vi "getSelectionValues.vi"(8 "error in (no error)":errorcluster, 11 "IProperty in":refnum<class "IProperty.lvclass">) -> (0 "error out":errorcluster, 2 "Selection Values out":refnum<class "IBaseObject.lvclass">, 3 "IProperty out":refnum<class "IProperty.lvclass">, 4 "Null?":bool)   [LabVIEW 2022 SP3, in "openDAQ.lvlib" / "IBaseObject.lvlib" / "IProperty.lvlib" / "IProperty.lvclass"]
uses:
  <instrlib>/openDAQ/Public/Classes/IProperty/IProperty.lvclass
  C:/Program Files (x86)/National Instruments/LabVIEW 2022/instr.lib/openDAQ/Public/Classes/IBaseObject/IBaseObject.lvclass
  <instrlib>/openDAQ/Public/Classes/IBaseObject/IBaseObject.lvclass
  <instrlib>/openDAQ/Public/Classes/IBaseObject/IBaseObject.lvclass/IBaseObject.ctl
  <instrlib>/openDAQ/Public/Classes/IBaseObject/Accessor/Read reference.vi
  <instrlib>/openDAQ/Public/Classes/IBaseObject/Accessor/Write reference.vi
  <instrlib>/openDAQ/Public/Classes/IProperty/IProperty.lvclass/IProperty.ctl
  <instrlib>/openDAQ/Binaries/Windows/x86/copendaq32.dll
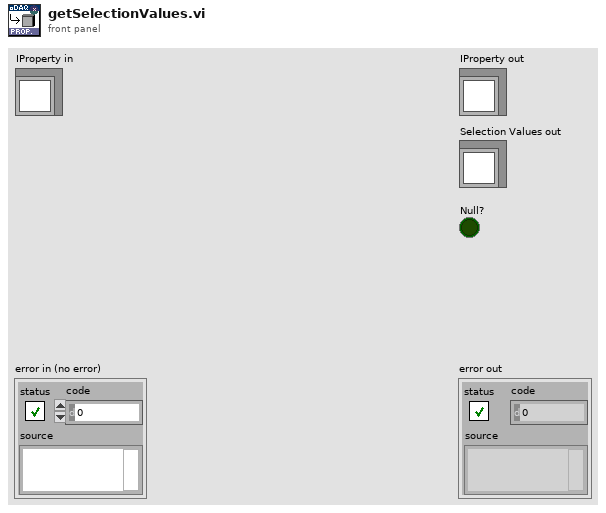
[diagram p1: front panel]
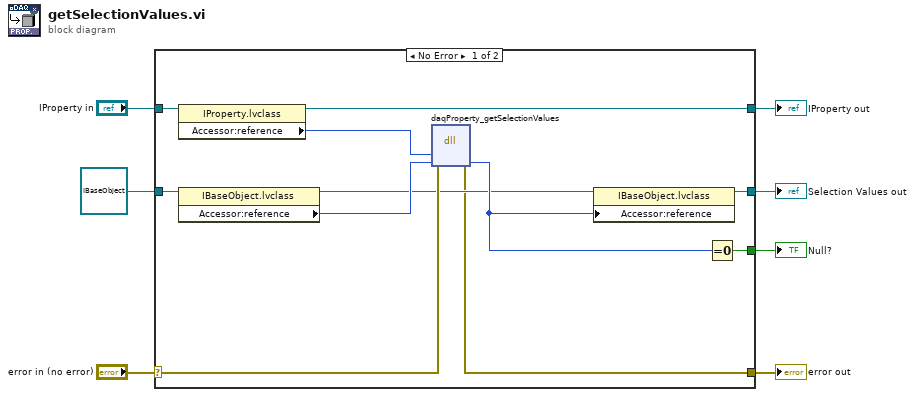
[diagram p0: block diagram]
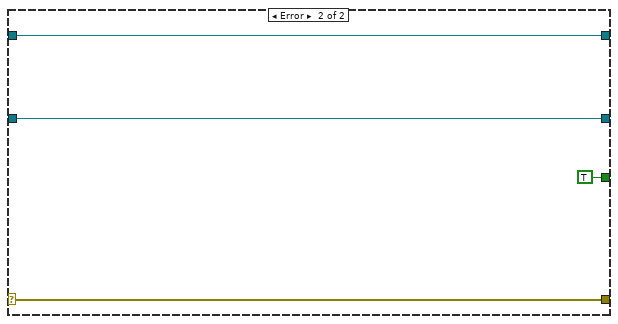
[diagram p2: hidden frame]
diagram:
  n1 = case shown="No Error" "error in (no error)" {
    selector: "error in (no error)" -> [w16 w22]
    tunnel: [w8 w22] -> w6
    tunnel: [w12 w21] -> w4
    tunnel: "IProperty in" -> [w17 w21]
    tunnel: refnum<class "IBaseObject.lvclass"> refnum ("openDAQ.lvlib:IBaseObject.lvlib:IBaseObject.lvclass") -> [w15 w20]
    tunnel: [w9 w20] -> w3
    tunnel: [w10 TRUE] -> w2
    frame No Error {
      n2 = property class="IProperty.lvclass"(reference=w17) -> (reference out=w12:refnum<class "IProperty.lvclass">, "Accessor:reference"=w14:i64)  [unwired: 1 in, 1 out]
      n3 = property class="IBaseObject.lvclass"(reference=w15) -> (reference out=w11:refnum<class "IBaseObject.lvclass">, "Accessor:reference"=w13:i64)  [unwired: 1 in, 1 out]
      n4 = dll-call lib="C:/Program Files (x86)/National Instruments/LabVIEW 2022/instr.lib/openDAQ/Binaries/Windows/x86/copendaq*.*" fn="daqProperty_getSelectionValues"(error in=w16, "property"=w14, "selectionValues"=w13) -> (error out=w8:errorcluster, "selectionValues"=w18:i64)  [unwired: 4 in, 1 out]
      n5 = property class="IBaseObject.lvclass"(reference=w11, "Accessor:reference"=w18) -> (reference out=w9:refnum<class "IBaseObject.lvclass">)  [unwired: 1 in, 1 out]
      n6 = Equal To 0?(x=w18) -> (x = 0?=w10:bool)
    }
    frame Error {
    }
  }
  "error out" <- w6
  "IProperty out" <- w4
  "Selection Values out" <- w3
  "Null?" <- w2
